vi "Set Vantage Lat V.vi"(8 "error in (no error)":errorcluster, 11 "latitude":T1) -> (0 "error out":errorcluster, 2 "function return":i16, 3 "latitude out":T1)   [LabVIEW 2009, in "VantagePro.lvlib"]
doc: "DllAccess short int _stdcall SetVantageLat_V ( LatLonValue *latitude);"
uses:
  VantagePro.lvlib
  <userlib>/VantagePro/VantagePro.dll
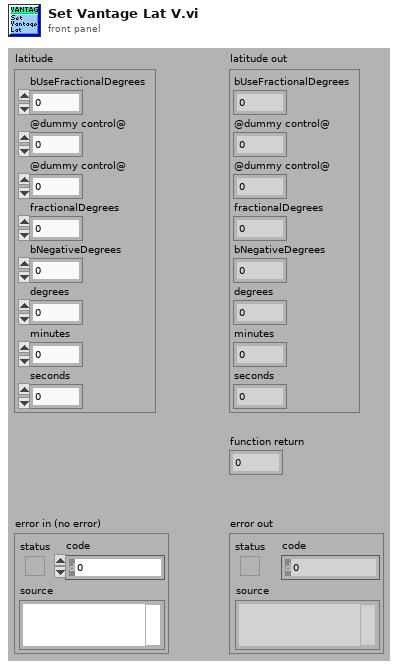
[diagram p1: front panel]
types:
  T1 = cluster{"bUseFractionalDegrees":i16, "@dummy control@":i8, "@dummy control@":i8, "fractionalDegrees":sgl, "bNegativeDegrees":i16, "degrees":i16, "minutes":i16, "seconds":i16}
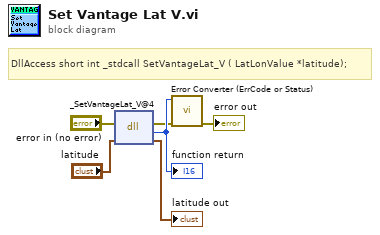
[diagram p0: block diagram]
diagram:
  # "DllAccess short int _stdcall SetVantageLat_V ( LatLonValue *latitude);"
  n1 = dll-call lib="C:/Program Files/National Instruments/LabVIEW 2010/user.lib/VantagePro/VantagePro.*" fn="_SetVantageLat_V@4"(error in="error in (no error)", "latitude"="latitude") -> (error out=w2:errorcluster, w6:i16, "latitude"=→"latitude out":T1)  [unwired: 2 in, 1 out]
  "function return" <- w6
  n2 = call "Error Converter (ErrCode or Status).vi"("error in (no error)"=w2, "error code"=w6) -> ("error out"=→"error out":errorcluster)  [unwired: 9 in]
